vi "enumerate subitems.vi"(11 "data to enumerate":string) -> (1 "associated data":string[](array[string]), 2 "discovered subitems":string[](array[string]), 3 "data out":string)   [LabVIEW 2013, in "TBM configuration.lvclass"]
doc: "Takes a set of wrapped data items and enumerates them. For example, the string:\n<a>s1</a>\n<b>s2</b>\nWill generate two lists containing [a,b] and [s1,s2]."
uses:
  TBM configuration.lvclass
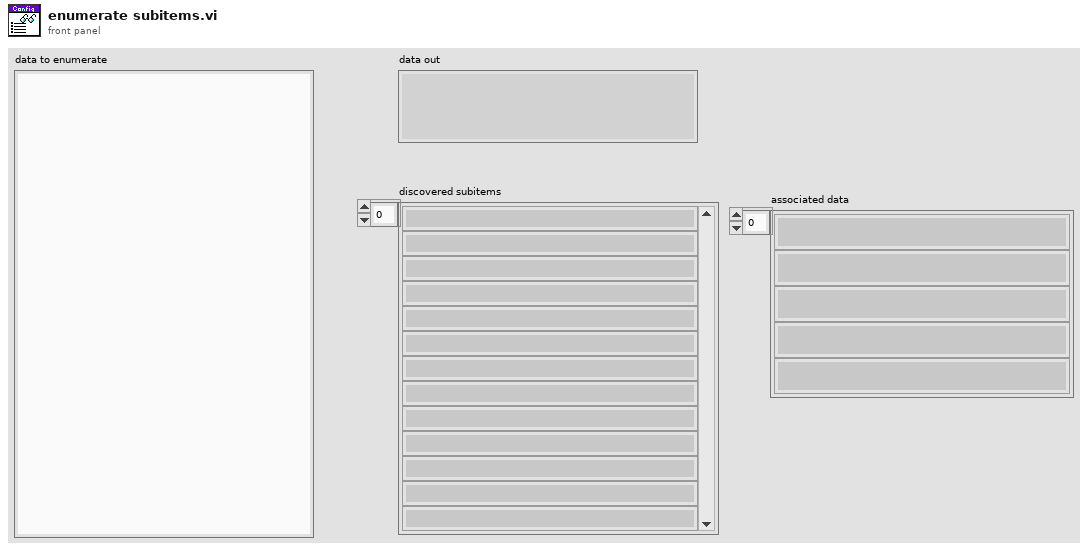
[diagram p1: front panel]
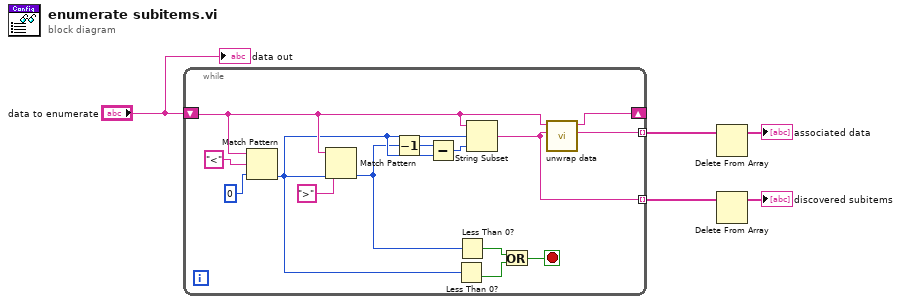
[diagram p0: block diagram]
diagram:
  n1 = while {
    shift-right: [w13] -> _
    shift-left: "data to enumerate" -> [w17]
    tunnel: [w12] -> w1 mode=indexing
    tunnel: [w11] -> w4 mode=indexing
    stop <- w14 stop-if-true
    n2 = Match Pattern(string=w17, regular expression="<", offset (0)=0) -> (offset past match=w9:i32)  [unwired: 3 out]
    n3 = Match Pattern(string=w17, regular expression=">", offset (0)=w9) -> (offset past match=w7:i32)  [unwired: 3 out]
    n4 = Decrement(x=w7) -> (x-1=w8:i32)
    n5 = Subtract(x=w8, y=w9) -> (x-y=w10:i32)
    n6 = Less Than 0?(x=w9) -> (x < 0?=w16:bool)
    n7 = Less Than 0?(x=w7) -> (x < 0?=w15:bool)
    n8 = String Subset(string=w17, offset (0)=w9, length (rest)=w10) -> (substring=w12:string)
    n9 = Or(x=w15, y=w16) -> (x .or. y?=w14:bool)
    n10 = call "unwrap data.vi"("identifier"=w12, "data to unwrap"=w17) -> ("unwrapped data"=w11:string, "remaining string"=w13:string)  [unwired: 8 in]
  }
  n11 = Delete From Array(array=w4) -> (array with subset deleted=→"associated data":string[])  [unwired: 2 in, 1 out]
  n12 = Delete From Array(array=w1) -> (array with subset deleted=→"discovered subitems":string[])  [unwired: 2 in, 1 out]
  "data out" <- "data to enumerate"
